vi "AI_alarm_Clusters_Sort_to_Numerics.vi"(11 "AllErrorStatus":T2) -> (3 "AI_Error_#s":T1)   [LabVIEW 2018]
uses:
  Controls/Clusts/All_AI_Error_Status.ctl
  Controls/Clusts/ErrorStatus.ctl
  Controls/Clusts/AI_Clust.ctl
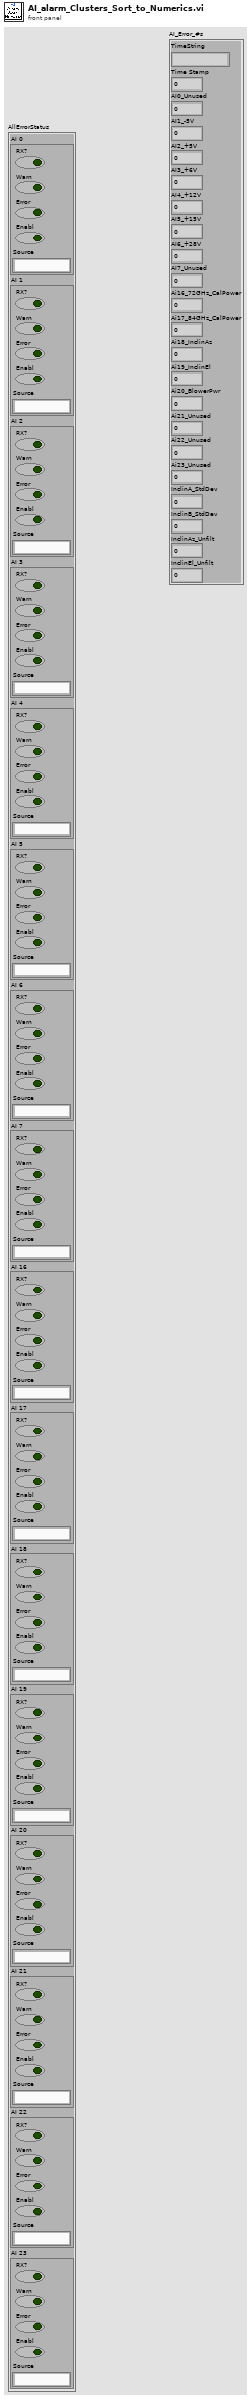
[diagram p1: front panel]
types:
  T1 = typedef "AI_Clust.ctl" = cluster{"TimeString":string, "Time Stamp":dbl, "AI0_Unused":dbl, "AI1_-5V":dbl, "AI2_+5V":dbl, "AI3_+6V":dbl, "AI4_+12V":dbl, "AI5_+15V":dbl, "AI6_+28V":dbl, "AI7_Unused":dbl, "Ai16_72GHz_CalPower":dbl, "Ai17_84GHz_CalPower":dbl, "Ai18_InclinAz":dbl, "Ai19_InclinEl":dbl, "Ai20_BlowerPwr":dbl, "Ai21_Unused":dbl, "Ai22_Unused":dbl, "Ai23_Unused":dbl, "InclinA_StdDev":dbl, "InclinB_StdDev":dbl, "InclinAz_Unfilt":dbl, "InclinEl_Unfilt":dbl}
  T2 = typedef "All_AI_Error_Status.ctl" = cluster{"AI 0":T3, "AI 1":T3, "AI 2":T3, "AI 3":T3, "AI 4":T3, "AI 5":T3, "AI 6":T3, "AI 7":T3, "AI 16":T3, "AI 17":T3, "AI 18":T3, "AI 19":T3, "AI 20":T3, "AI 21":T3, "AI 22":T3, "AI 23":T3}
  T3 = typedef "ErrorStatus.ctl" = cluster{"RX?":bool, "Warn":bool, "Error":bool, "Enabl":bool, "Source":string}
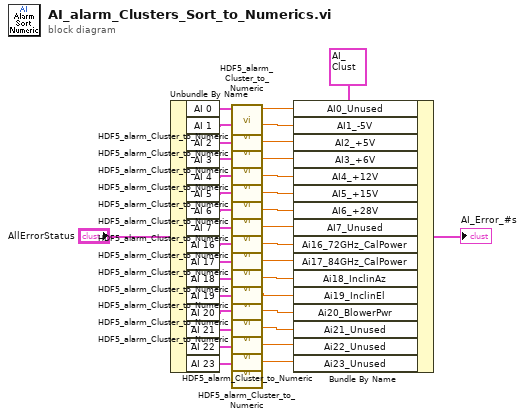
[diagram p0: block diagram]
diagram:
  n1 = Unbundle By Name("AllErrorStatus") -> ("AI 0"=w34:T3, "AI 1"=w19:T3, "AI 2"=w20:T3, "AI 3"=w21:T3, "AI 4"=w22:T3, "AI 5"=w23:T3, "AI 6"=w24:T3, "AI 7"=w25:T3, "AI 16"=w26:T3, "AI 17"=w27:T3, "AI 18"=w28:T3, "AI 19"=w29:T3, "AI 20"=w30:T3, "AI 21"=w31:T3, "AI 22"=w32:T3, "AI 23"=w33:T3)
  n2 = call "HDF5_alarm_Cluster_to_Numeric.vi"("TC 0"=w34) -> ("f"=w35:dbl)  [unwired: 10 in]
  n3 = call "HDF5_alarm_Cluster_to_Numeric.vi"("TC 0"=w19) -> ("f"=w18:dbl)  [unwired: 10 in]
  n4 = call "HDF5_alarm_Cluster_to_Numeric.vi"("TC 0"=w20) -> ("f"=w17:dbl)  [unwired: 10 in]
  n5 = call "HDF5_alarm_Cluster_to_Numeric.vi"("TC 0"=w21) -> ("f"=w16:dbl)  [unwired: 10 in]
  n6 = call "HDF5_alarm_Cluster_to_Numeric.vi"("TC 0"=w22) -> ("f"=w15:dbl)  [unwired: 10 in]
  n7 = call "HDF5_alarm_Cluster_to_Numeric.vi"("TC 0"=w23) -> ("f"=w14:dbl)  [unwired: 10 in]
  n8 = call "HDF5_alarm_Cluster_to_Numeric.vi"("TC 0"=w24) -> ("f"=w13:dbl)  [unwired: 10 in]
  n9 = call "HDF5_alarm_Cluster_to_Numeric.vi"("TC 0"=w25) -> ("f"=w12:dbl)  [unwired: 10 in]
  n10 = call "HDF5_alarm_Cluster_to_Numeric.vi"("TC 0"=w26) -> ("f"=w11:dbl)  [unwired: 10 in]
  n11 = call "HDF5_alarm_Cluster_to_Numeric.vi"("TC 0"=w27) -> ("f"=w10:dbl)  [unwired: 10 in]
  n12 = call "HDF5_alarm_Cluster_to_Numeric.vi"("TC 0"=w28) -> ("f"=w9:dbl)  [unwired: 10 in]
  n13 = call "HDF5_alarm_Cluster_to_Numeric.vi"("TC 0"=w29) -> ("f"=w8:dbl)  [unwired: 10 in]
  n14 = call "HDF5_alarm_Cluster_to_Numeric.vi"("TC 0"=w30) -> ("f"=w7:dbl)  [unwired: 10 in]
  n15 = call "HDF5_alarm_Cluster_to_Numeric.vi"("TC 0"=w31) -> ("f"=w6:dbl)  [unwired: 10 in]
  n16 = call "HDF5_alarm_Cluster_to_Numeric.vi"("TC 0"=w32) -> ("f"=w5:dbl)  [unwired: 10 in]
  n17 = call "HDF5_alarm_Cluster_to_Numeric.vi"("TC 0"=w33) -> ("f"=w4:dbl)  [unwired: 10 in]
  n18 = Bundle By Name(cluster=T1 {"TimeString"="", "Time Stamp"=0.0, "AI0_Unused"=0.0, "AI1_-5V"=0.0, "AI2_+5V"=0.0, "AI3_+6V"=0.0, "AI4_+12V"=0.0, "AI5_+15V"=0.0, "AI6_+28V"=0.0, "AI7_Unused"=0.0, "Ai16_72GHz_CalPower"=0.0, "Ai17_84GHz_CalPower"=0.0, "Ai18_InclinAz"=0.0, "Ai19_InclinEl"=0.0, "Ai20_BlowerPwr"=0.0, "Ai21_Unused"=0.0, "Ai22_Unused"=0.0, "Ai23_Unused"=0.0, "InclinA_StdDev"=0.0, "InclinB_StdDev"=0.0, "InclinAz_Unfilt"=0.0, "InclinEl_Unfilt"=0.0} ("AI"), "AI0_Unused"=w35, "AI1_-5V"=w18, "AI2_+5V"=w17, "AI3_+6V"=w16, "AI4_+12V"=w15, "AI5_+15V"=w14, "AI6_+28V"=w13, "AI7_Unused"=w12, "Ai16_72GHz_CalPower"=w11, "Ai17_84GHz_CalPower"=w10, "Ai18_InclinAz"=w9, "Ai19_InclinEl"=w8, "Ai20_BlowerPwr"=w7, "Ai21_Unused"=w6, "Ai22_Unused"=w5, "Ai23_Unused"=w4) -> (→"AI_Error_#s":T1)
